vi "S2C_XML_UpdateTestStatus.vi"(8 "Error In":errorcluster, 11 "Result":string) -> (0 "Error Out":errorcluster)   [LabVIEW 2015]
uses:
  S2C_XML_Globals.vi
  <vilib>/xml/Close Reference(Node).vi
  <resource>/objmgr/DOMUserDefRef.rc
  <vilib>/xml/NI_XML.lvlib
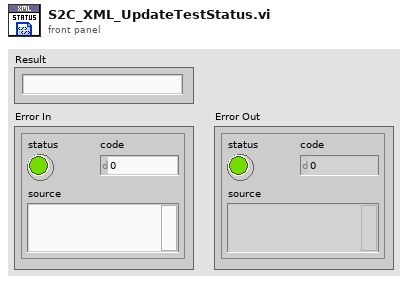
[diagram p1: front panel]
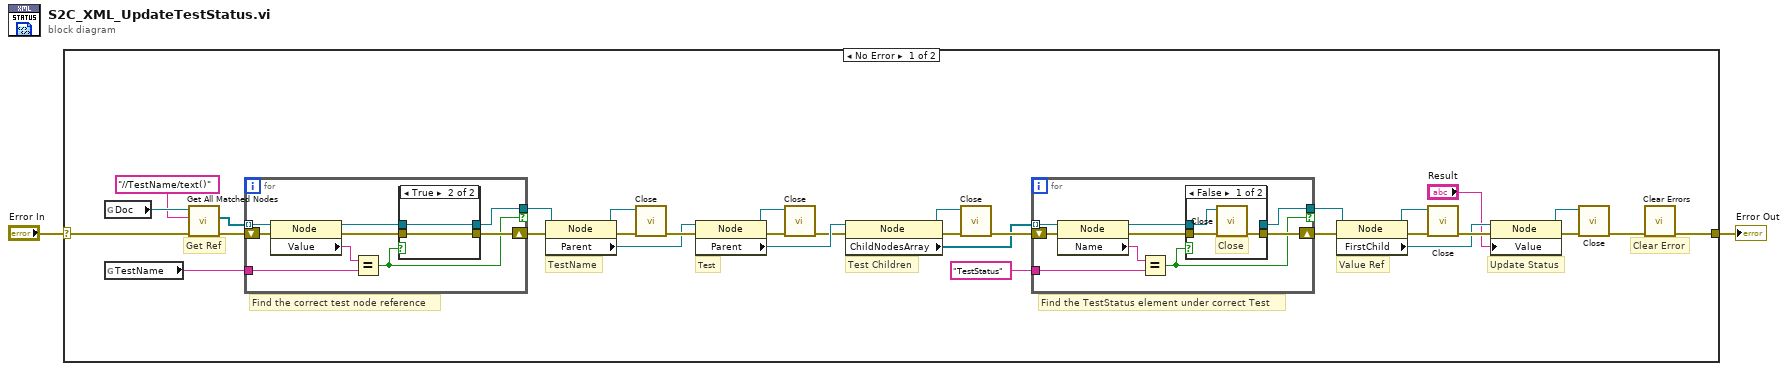
[diagram p0: block diagram]
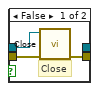
[diagram p3: hidden frame]
diagram:
  n1 = case shown="No Error" "Error In" {
    selector: "Error In" -> [w32 w63]
    tunnel: [w3 w63] -> w2
    frame No Error {
      # "Clear Error"
      # "Update Status"
      # "Value Ref"
      # "Find the TestStatus element under correct Test"
      # "Test Children"
      # "Test"
      # "TestName"
      # "Find the correct test node reference"
      # "Get Ref"
      n2 = global read "S2C_XML_Globals.vi" "Doc"() -> (w34:refnum<k20>)
      n3 = global read "S2C_XML_Globals.vi" "TestName"() -> (w30:string)
      n4 = call <vilib>:"Get All Matched Nodes.vi"("error in (no error)"=w32, "XPath expression"="//TestName/text()", "node in"=w34) -> ("error out"=w33:errorcluster, "node result array"=w31:refnum<k20>[])  [unwired: 6 in, 1 out]
      n5 = for {
        tunnel: w31 -> [w56] mode=indexing
        tunnel: w30 -> [w54]
        shift-right: [w51] -> w29
        shift-left: w33 -> [w57]
        tunnel: [w50] -> w28 if=w49
        n6 = property class="Node"(reference=w56, error in=w57) -> (reference out=w52:refnum<k20>, error out=w53:errorcluster, "Value"=w55:string)
        n7 = Equal?(x=w55, y=w54) -> (x = y?=w49:bool)
        n8 = case shown="True" w49 {
          tunnel: w53 -> [w60 w62]
          tunnel: w52 -> [w59 w61]
          tunnel: [w58 w62] -> w51
          tunnel: [_ w61] -> w50
          frame False {
            # "Close"
            n9 = call-poly <vilib>:"Close.vi"("error in (no error)"=w60, "node"=w59) -> ("error out"=w58:errorcluster)  [unwired: 7 in]
          }
          frame True {
          }
        }
      }
      n10 = property class="Node"(reference=w28, error in=w29) -> (reference out=w26:refnum<k20>, error out=w27:errorcluster, "Parent"=w24:refnum<k20>)
      n11 = call-poly <vilib>:"Close.vi"("error in (no error)"=w27, "node"=w26) -> ("error out"=w25:errorcluster)  [unwired: 7 in]
      n12 = property class="Node"(reference=w24, error in=w25) -> (reference out=w22:refnum<k20>, error out=w23:errorcluster, "Parent"=w21:refnum<k20>)
      n13 = call-poly <vilib>:"Close.vi"("error in (no error)"=w23, "node"=w22) -> ("error out"=w20:errorcluster)  [unwired: 7 in]
      n14 = property class="Node"(reference=w21, error in=w20) -> (reference out=w18:refnum<k20>, error out=w19:errorcluster, "ChildNodesArray"=w6:refnum<k20>[])
      n15 = call-poly <vilib>:"Close.vi"("error in (no error)"=w19, "node"=w18) -> ("error out"=w9:errorcluster)  [unwired: 7 in]
      n16 = for {
        tunnel: w6 -> [w42] mode=indexing
        tunnel: "TestStatus" ("Node Value") -> [w40]
        shift-right: [w37] -> w8
        shift-left: w9 -> [w43]
        tunnel: [w36] -> w7 if=w35
        n17 = property class="Node"(reference=w42, error in=w43) -> (reference out=w38:refnum<k20>, error out=w39:errorcluster, "Name"=w41:string)
        n18 = Equal?(x=w41, y=w40) -> (x = y?=w35:bool)
        n19 = case shown="False" w35 {
          tunnel: w39 -> [w46 w48]
          tunnel: w38 -> [w45 w47]
          tunnel: [w44 w48] -> w37
          tunnel: [_ w47] -> w36
          frame False {
            # "Close"
            n20 = call-poly <vilib>:"Close.vi"("error in (no error)"=w46, "node"=w45) -> ("error out"=w44:errorcluster)  [unwired: 7 in]
          }
          frame True {
          }
        }
      }
      n21 = property class="Node"(reference=w7, error in=w8) -> (reference out=w16:refnum<k20>, error out=w17:errorcluster, "FirstChild"=w14:refnum<k20>)
      n22 = call-poly <vilib>:"Close.vi"("error in (no error)"=w17, "node"=w16) -> ("error out"=w15:errorcluster)  [unwired: 7 in]
      n23 = property class="Node"(reference=w14, error in=w15, "Value"="Result") -> (reference out=w12:refnum<k20>, error out=w13:errorcluster)
      n24 = call-poly <vilib>:"Close.vi"("error in (no error)"=w13, "node"=w12) -> ("error out"=w4:errorcluster)  [unwired: 7 in]
      n25 = call <vilib>:"Clear Errors.vi"("error in (no error)"=w4) -> ("error out"=w3:errorcluster)  [unwired: 5 in, 1 out]
    }
    frame Error {
    }
  }
  "Error Out" <- w2
